vi "linx_stepper_control.vi"() -> ()   [LabVIEW 2017]
uses:
  <vilib>/MakerHub/LINX/Public/Peripherals/Digital/Digital Read 1 Chan.vi
  <vilib>/MakerHub/LINX/Public/Peripherals/Digital/Digital Read N Chans.vi
  <vilib>/MakerHub/LINX/Private/Local IO/LinxDigitalRead.vi
  <vilib>/MakerHub/LINX/Public/Utilities/Check Channel.vi
  <vilib>/MakerHub/LINX/Public/Utilities/Open Serial.vi
  <vilib>/MakerHub/LINX/Private/Utilties/Generate Error.vi
  <vilib>/MakerHub/LINX/LMH-LINX.lvlib
panel:
  out "position":sgl[unit] format="%#.6g"
  in  "home stepper":bool
  in  "error in (no error)":errorcluster
  in  "MG17Motor":refnum<k7>(container)
  out "counter":dbl
  out "up/down/same":i32
  out "Response encoder signed long":sgl
  out "Response i2c":u8[](array[numeric])
  in  "Line 1":string
  in  "Line 0":string
  out "step size":dbl
  out "DI Value":bool
  in  "stop":bool
  out "Response encoder":u8[](array[numeric])
  in  "Timeout (100 ms)":i32=100
  in  "Serial Port":refnum<visa-resource-name>="COM4"
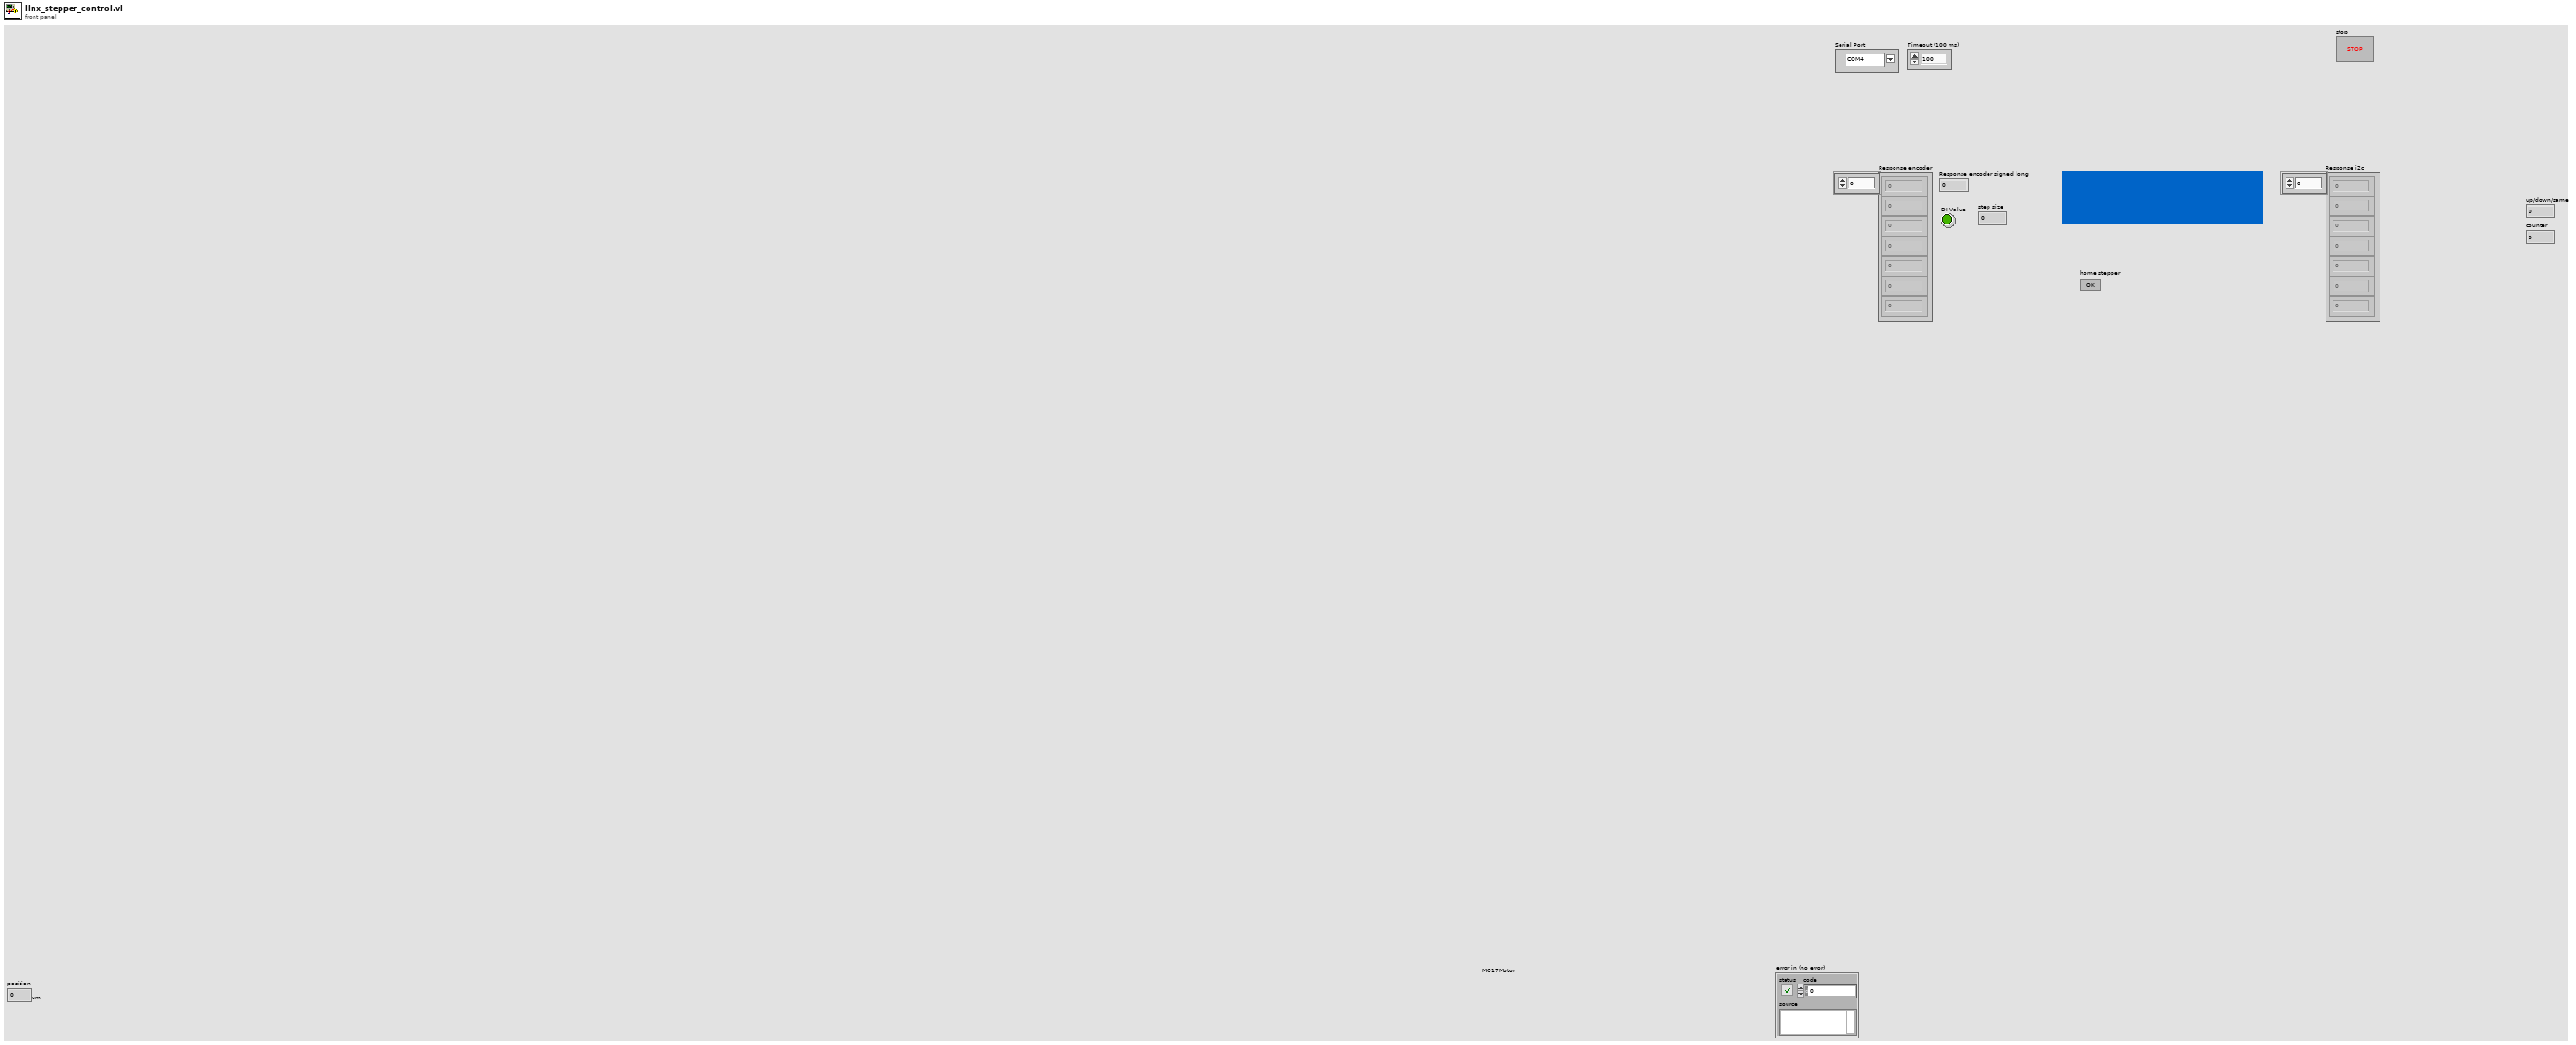
[diagram p1: front panel]
types:
  T1 = typedef "LMH-LINX.lvlib/LINX Ref.ctl" = cluster{"IO":T2, "Interface":T3, "LINX Device Config":T4}
  T2 = typedef "LMH-LINX.lvlib/Platform.ctl" = enum16{"Remote", "Local"}
  T3 = typedef "LMH-LINX.lvlib/Interface.ctl" = enum16{"Serial", "TCP"}
  T4 = typedef "LMH-LINX.lvlib/Device.lvlib/LINX Device Config.ctl" = cluster{"Interface":T3, "COM Port":refnum<visa-resource-name>, "TCP Configuration":T5, "Device Family":u8, "Device ID":u8, "Device Name":string, "TCP Ref":refnum<k5>, "Channels":T6}
  T5 = typedef "LMH-LINX.lvlib/Device.lvlib/TCP Config.ctl" = cluster{"IP Address":string, "Port":u16}
  T6 = typedef "LMH-LINX.lvlib/Channels.ctl" = cluster{"DI":u8[], "DO":u8[], "AI":u8[], "AO":u8[], "PWM":u8[], "QE":u8[], "UART":u8[], "I2C 2":u8[], "SPI":u8[], "CAN":u8[], "Servo":u8[], "AI Ref (V)":dbl, "AI Resolution (Bits)":u8, "AO Ref (V)":dbl, "AO Resolution (Bits)":u8}
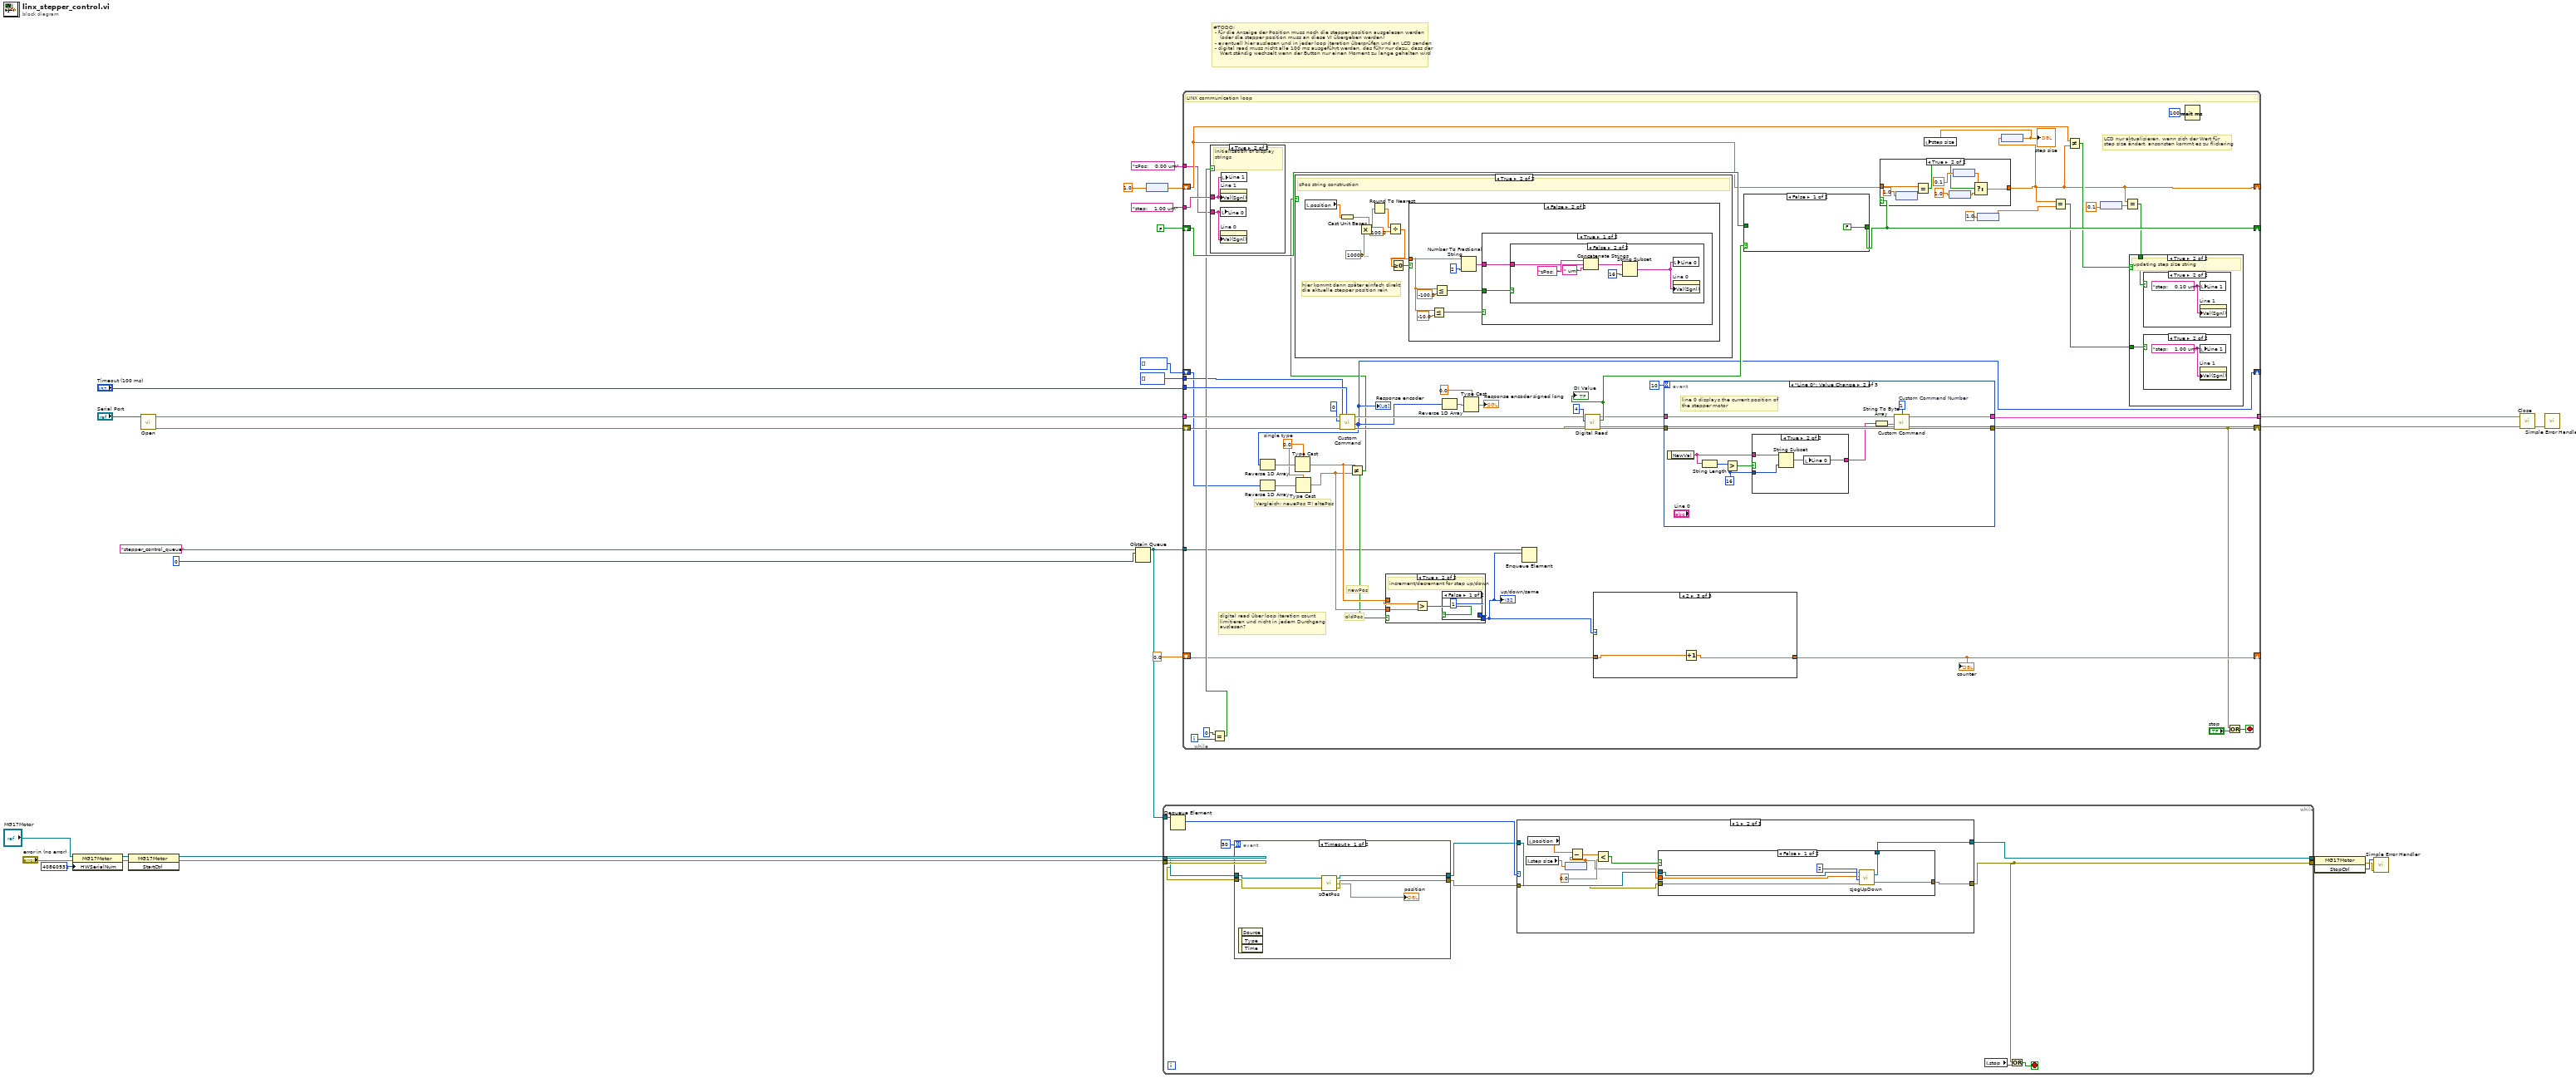
[diagram p0: block diagram]
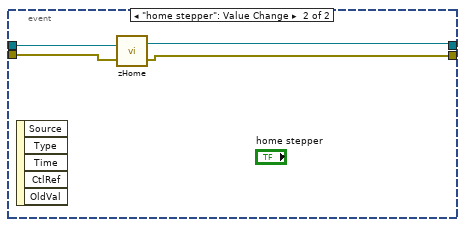
[diagram p2: hidden frame]
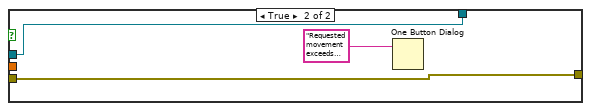
[diagram p4: hidden frame]
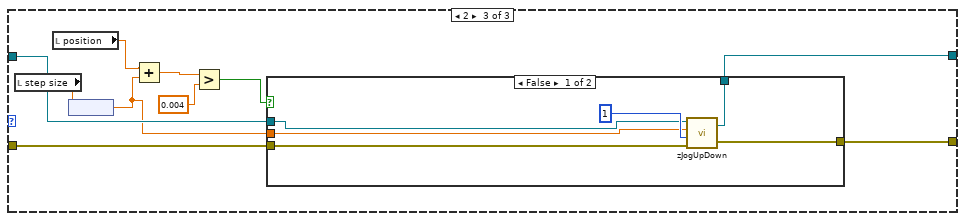
[diagram p5: hidden frame]
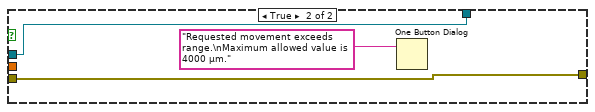
[diagram p6: hidden frame]
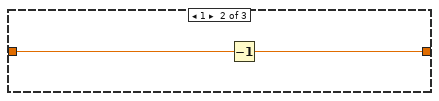
[diagram p8: hidden frame]
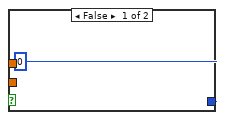
[diagram p9: hidden frame]
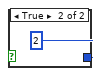
[diagram p10: hidden frame]
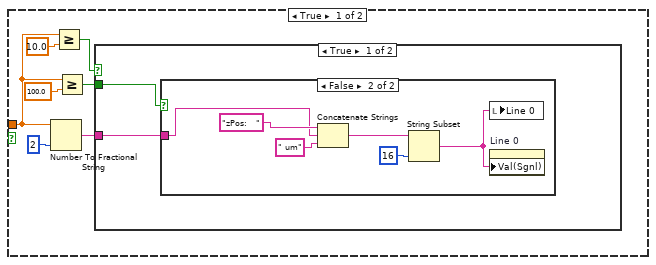
[diagram p12: hidden frame]
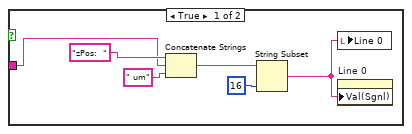
[diagram p13: hidden frame]
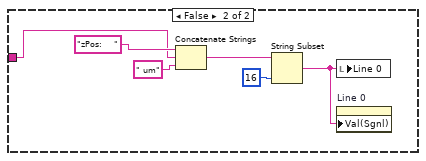
[diagram p14: hidden frame]
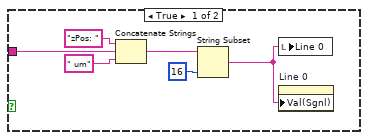
[diagram p15: hidden frame]
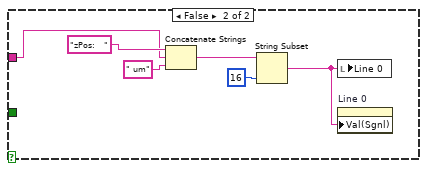
[diagram p16: hidden frame]
diagram:
  # "#TODO:\n - für die Anzeige der Position muss noch die stepper position ausgelesen werden\n    (oder die stepper position muss an diese VI übergeben werden)\n - eventuell hier auslesen und in jeder loop iteration überprüfen und an LCD senden\n - digital read muss nicht alle 100 ms ausgeführt werden, das führ nur dazu, dass der \n    Wert ständig wechselt wenn der Button nur einen Moment zu lange gehalten wird"
  n1 = property class="MG17Motor"(reference="MG17Motor", error in="error in (no error)", "HWSerialNum"=40860931) -> (reference out=w16:refnum<k7>, error out=w13:errorcluster)
  n2 = invoke class="MG17Motor" method="StartCtrl"(reference=w16, error in=w13) -> (reference out=w11:refnum<k7>, error out=w10:errorcluster)  [unwired: 1 in, 1 out]
  n3 = call-poly <vilib>:"Open.vi"("Serial Port"="Serial Port") -> ("Error Out"=w28:errorcluster, "LINX Resource"=w27:T1)  [unwired: 8 in, 1 out]
  n4 = Obtain Queue(name (unnamed)="stepper_control_queue", element data type=0) -> (queue out=w3:refnum<queue>)  [unwired: 3 in, 2 out]
  n5 = node(1.0) -> (w1:dbl[unit])
  n6 = while {
    tunnel: w11 -> [w37]
    tunnel: w10 -> [w36]
    tunnel: [w33] -> w9
    tunnel: [w32] -> w8
    tunnel: w3 -> [w39]
    stop <- w40 stop-if-true
    n7 = Dequeue Element(queue=w39) -> (element=w38:i32)  [unwired: 2 in, 3 out]
    n8 = event shown="[0] Timeout" {
      selector: _ -> [_ _]
      dyn-events: _ -> [_ _]
      timeout: 50 -> [_ _]
      tunnel: w37 -> [w45 w49]
      tunnel: w36 -> [w44 w46]
      tunnel: [w43 w48] -> w35
      tunnel: [w42 w47] -> w34
      event Timeout {
        n9 = event-data() -> ()  [unwired: 1 in, 3 out]
        n10 = call "zGetPos.vi"("error in (no error)"=w44, "reference in"=w45) -> ("error out"=w42:errorcluster, "position"=→"position":sgl[unit], "reference out"=w43:refnum<k7>)  [unwired: 1 in]
      }
      event "home stepper": Value Change {
        n11 = event-data() -> ()  [unwired: 1 in, 5 out]
        n12 = call "zHome.vi"("error in"=w46, "reference in"=w49) -> ("error out"=w47:errorcluster, "reference out"=w48:refnum<k7>)
      }
    }
    n13 = case shown="1" w38 {
      tunnel: w35 -> [w51 w55 w80]
      tunnel: w34 -> [w50 w54 w79]
      tunnel: [w51 w52 w78] -> w33
      tunnel: [w50 w53 w77] -> w32
      frame 0, Default {
      }
      frame 1 {
        n14 = local read "step size"() -> (w57:dbl)
        n15 = local read "position"() -> (w59:sgl[unit])
        n16 = node(w57) -> (w56:dbl[unit])
        n17 = Subtract(x=w59, y=w56) -> (x-y=w60:dbl[unit])
        n18 = Less?(x=w60, y=sgl[unit] 0.0) -> (x < y?=w58:bool)
        n19 = case shown="False" w58 {
          tunnel: [w67 w69] -> w53
          tunnel: w56 -> [w65 _]
          tunnel: w55 -> [w64 w68]
          tunnel: w54 -> [w63 w69]
          tunnel: [w62 w68] -> w52
          frame False {
            n20 = call "zJogUpDown.vi"("error in"=w63, "lJogDir"=2, "fStepSize"=w65, "reference in"=w64) -> ("error out"=w67:errorcluster, "reference out"=w62:refnum<k7>)
          }
          frame True {
            n21 = One Button Dialog(message="Requested movement exceeds range.\nMinimum allowed value is 0 µm.") -> ()  [unwired: 1 in, 1 out]
          }
        }
      }
      frame 2 {
        n22 = local read "step size"() -> (w72:dbl)
        n23 = local read "position"() -> (w73:sgl[unit])
        n24 = node(w72) -> (w71:dbl[unit])
        n25 = Add(x=w73, y=w71) -> (x+y=w75:dbl[unit])
        n26 = Greater?(x=w75, y=dbl[unit] 0.004) -> (0:w74:bool)
        n27 = case shown="False" w74 {
          tunnel: [w86 w88] -> w77
          tunnel: w71 -> [w81 _]
          tunnel: w80 -> [w84 w87]
          tunnel: w79 -> [w83 w88]
          tunnel: [w82 w87] -> w78
          frame False {
            n28 = call "zJogUpDown.vi"("error in"=w83, "lJogDir"=1, "fStepSize"=w81, "reference in"=w84) -> ("error out"=w86:errorcluster, "reference out"=w82:refnum<k7>)
          }
          frame True {
            n29 = One Button Dialog(message="Requested movement exceeds range.\nMaximum allowed value is 4000 µm.") -> ()  [unwired: 1 in, 1 out]
          }
        }
      }
    }
    n30 = local read "stop"() -> (w30:bool)
    n31 = Or(x=w32, y=w30) -> (x .or. y?=w40:bool)
  }
  n32 = while {
    tunnel: "Timeout (100 ms)" -> [w136]
    shift-right: [w96] -> w26
    shift-left: w28 -> [w138]
    shift-right: [w107] -> _
    shift-left: u8[] [] ("Response") -> [w104]
    tunnel: w27 -> [w137]
    tunnel: [w127] -> w25
    shift-right: [w91] -> _
    shift-left: w1 -> [w122]
    shift-right: [w130] -> _
    shift-left: FALSE -> [w131]
    tunnel: "step:    1,00 um" -> [w121]
    tunnel: "zPos:    0,00 um" -> [w113]
    tunnel: u8[] [] ("Data") -> [w112]
    shift-right: [w99] -> _
    shift-left: 0.0 -> [w100]
    tunnel: w3 -> [w98]
    i -> [w120]
    stop <- w134 stop-if-true
    w105 = sgl 0.0  # single type
    # "oldPos"
    # "newPos"
    # "Vergleich: neuePos =! altePos"
    # "LCD nur aktualisieren, wenn sich der Wert für\nstep size ändert, ansonsten kommt es zu flickering"
    # "digital read über loop iteration count \nlimitieren und nicht in jedem Durchgang \nauslesen?"
    # "LINX communication loop"
    n33 = Equal?(x=0, y=w120) -> (x = y?=w118:bool)
    n34 = case shown="True" w118 {
      tunnel: w121 -> [_ w214]
      tunnel: w113 -> [_ w213]
      frame False {
      }
      frame True {
        # "initialization of display strings"
        n35 = property on="Line 1" class="Str"("Val(Sgnl)"=w214) -> ()  [unwired: 2 in, 2 out]
        n36 = local write "Line 0"(w213) -> ()
        n37 = property on="Line 0" class="Str"("Val(Sgnl)"=w213) -> ()  [unwired: 2 in, 2 out]
        n38 = local write "Line 1"(w214) -> ()
      }
    }
    n39 = Reverse 1D Array(array=w104) -> (reversed array=w106:u8[])
    n40 = Type Cast(type=w105, x=w106) -> (*(type *) &x=w102:sgl)
    n41 = call <vilib>:"Custom Command.vi"("Timeout (100 ms)"=w136, "Error In"=w138, "Data"=w112, "Custom Command Number"=u16 0, "LINX Resource"=w137) -> ("Error Out"=w116:errorcluster, "Response"=w107:u8[], "LINX Resource"=w117:T1)  [unwired: 3 in, 1 out]
    "Response encoder" <- w107
    n42 = Reverse 1D Array(array=w107) -> (reversed array=w108:u8[])
    n43 = Type Cast(type=w105, x=w108) -> (*(type *) &x=w103:sgl)
    n44 = Not Equal?(x=w103, y=w102) -> (x != y?=w101:bool)
    n45 = case shown="True" w101 {
      frame False {
      }
      frame True {
        # "hier kommt dann später einfach direkt\ndie aktuelle stepper position rein"
        # "zPos string construction"
        n46 = local read "position"() -> (w157:sgl[unit])
        n47 = Cast Unit Bases(0:w157) -> (2:w155:sgl)  [unwired: 1 in]
        n48 = Multiply(x=w155, y=sgl 100000000.0) -> (x*y=w154:sgl)
        n49 = Round To Nearest(number=w154) -> (nearest integer value=w153:sgl)
        n50 = Divide(x=w153, y=sgl 100.0) -> (x/y=w151:sgl)
        n51 = Greater Or Equal To 0?(x=w151) -> (x >= 0?=w158:bool)
        n52 = case shown="False" w158 {
          tunnel: w151 -> [w159 w188]
          frame True {
            n53 = Number To Fractional String(number=w159, precision (6)=i16 2) -> (F-format string=w160:string)  [unwired: 2 in]
            n54 = Greater Or Equal?(x=w159, y=sgl 10.0 ("x")) -> (x >= y?=w165:bool)
            n55 = Greater Or Equal?(x=w159, y=sgl 100.0 ("x")) -> (x >= y?=w162:bool)
            n56 = case shown="True" w165 {
              tunnel: w160 -> [w167 w180]
              tunnel: w162 -> [w166 _]
              frame True {
                n57 = case shown="False" w166 {
                  tunnel: w167 -> [w168 w174]
                  frame True {
                    n58 = Concatenate Strings("zPos:  ", w168, " um") -> (w172:string)
                    n59 = String Subset(string=w172, length (rest)=16 ("length (rest)")) -> (substring=w171:string)  [unwired: 1 in]
                    n60 = local write "Line 0"(w171) -> ()
                    n61 = property on="Line 0" class="Str"("Val(Sgnl)"=w171) -> ()  [unwired: 2 in, 2 out]
                  }
                  frame False {
                    n62 = Concatenate Strings("zPos:   ", w174, " um") -> (w178:string)
                    n63 = String Subset(string=w178, length (rest)=16 ("length (rest)")) -> (substring=w177:string)  [unwired: 1 in]
                    n64 = local write "Line 0"(w177) -> ()
                    n65 = property on="Line 0" class="Str"("Val(Sgnl)"=w177) -> ()  [unwired: 2 in, 2 out]
                  }
                }
              }
              frame False {
                n66 = Concatenate Strings("zPos:    ", w180, " um") -> (w184:string)
                n67 = String Subset(string=w184, length (rest)=16 ("length (rest)")) -> (substring=w183:string)  [unwired: 1 in]
                n68 = local write "Line 0"(w183) -> ()
                n69 = property on="Line 0" class="Str"("Val(Sgnl)"=w183) -> ()  [unwired: 2 in, 2 out]
              }
            }
          }
          frame False {
            n70 = Less Or Equal?(x=w188, y=sgl -10.0 ("x")) -> (x <= y?=w192:bool)
            n71 = Less Or Equal?(x=w188, y=sgl -100.0 ("x")) -> (x <= y?=w190:bool)
            n72 = Number To Fractional String(number=w188, precision (6)=i16 2) -> (F-format string=w187:string)  [unwired: 2 in]
            n73 = case shown="True" w192 {
              tunnel: w190 -> [w194 _]
              tunnel: w187 -> [w193 w207]
              frame True {
                n74 = case shown="False" w194 {
                  tunnel: w193 -> [w195 w201]
                  frame True {
                    n75 = Concatenate Strings("zPos: ", w195, " um") -> (w199:string)
                    n76 = String Subset(string=w199, length (rest)=16 ("length (rest)")) -> (substring=w198:string)  [unwired: 1 in]
                    n77 = local write "Line 0"(w198) -> ()
                    n78 = property on="Line 0" class="Str"("Val(Sgnl)"=w198) -> ()  [unwired: 2 in, 2 out]
                  }
                  frame False {
                    n79 = Concatenate Strings("zPos:  ", w201, " um") -> (w205:string)
                    n80 = String Subset(string=w205, length (rest)=16 ("length (rest)")) -> (substring=w204:string)  [unwired: 1 in]
                    n81 = local write "Line 0"(w204) -> ()
                    n82 = property on="Line 0" class="Str"("Val(Sgnl)"=w204) -> ()  [unwired: 2 in, 2 out]
                  }
                }
              }
              frame False {
                n83 = Concatenate Strings("zPos:   ", w207, " um") -> (w211:string)
                n84 = String Subset(string=w211, length (rest)=16 ("length (rest)")) -> (substring=w210:string)  [unwired: 1 in]
                n85 = local write "Line 0"(w210) -> ()
                n86 = property on="Line 0" class="Str"("Val(Sgnl)"=w210) -> ()  [unwired: 2 in, 2 out]
              }
            }
          }
        }
      }
    }
    n87 = case shown="True" w101 {
      tunnel: w103 -> [_ w148]
      tunnel: w102 -> [_ w147]
      tunnel: [0 w145] -> w97
      frame False {
      }
      frame True {
        # "increment/decrement for step up/down"
        n88 = Greater?(x=w148, y=w147) -> (0:w146:bool)
        n89 = case shown="False" w146 {
          tunnel: [1 2] -> w145
          frame False {
          }
          frame True {
          }
        }
      }
    }
    "up/down/same" <- w97
    n90 = Reverse 1D Array(array=w107) -> (reversed array=w111:u8[])
    n91 = Type Cast(type=sgl 0.0, x=w111) -> (*(type *) &x=→"Response encoder signed long":sgl)
    n92 = Enqueue Element(queue=w98, element=w97) -> ()  [unwired: 2 in, 3 out]
    n93 = call-poly <vilib>:"Digital Read.vi"("Error In"=w116, "DI Channel"=u8 4, "LINX Resource"=w117) -> ("Error Out"=w128:errorcluster, "DI Value"=w132:bool, "LINX Resource"=w129:T1)  [unwired: 6 in]
    "DI Value" <- w132
    n94 = case shown="2" w97 {
      tunnel: w100 -> [w139 w141 w143]
      tunnel: [w139 w140 w142] -> w99
      frame 0, Default {
      }
      frame 1 {
        n95 = Decrement(x=w141) -> (x-1=w140:dbl)
      }
      frame 2 {
        n96 = Increment(x=w143) -> (x+1=w142:dbl)
      }
    }
    "counter" <- w99
    n97 = event shown="[1] \"Line 0\": Value Change" {
      selector: _ -> [_ _ _]
      dyn-events: _ -> [_ _ _]
      timeout: 10 -> [_ _ _]
      tunnel: w129 -> [w219 w227 w243]
      tunnel: [w219 w225 w241] -> w127
      tunnel: [w220 w224 w240] -> w96
      tunnel: w128 -> [w220 w226 w242]
      event Timeout {
        n98 = event-data() -> ()  [unwired: 1 in, 1 out]
      }
      event "Line 0": Value Change {
        w221 = u16 1  # Custom Command Number
        w228 = 16 ("y")
        # "line 0 displays the current position of \nthe stepper motor"
        n99 = event-data() -> ("NewVal"=w229:string)  [unwired: 1 in]
        n100 = String Length(string=w229) -> (length=w231:i32)
        n101 = Greater?(x=w231, y=w228) -> (0:w230:bool)
        n102 = case shown="True" w230 {
          tunnel: w229 -> [w232 w235]
          tunnel: w228 -> [_ w234]
          tunnel: [w232 w233] -> w222
          frame False {
          }
          frame True {
            n103 = String Subset(string=w235, length (rest)=w234) -> (substring=w233:string)  [unwired: 1 in]
            n104 = local write "Line 0"(w233) -> ()
          }
        }
        n105 = String To Byte Array(string=w222) -> (unsigned byte array=w223:u8[])
        n106 = call <vilib>:"Custom Command.vi"("Error In"=w226, "Data"=w223, "Custom Command Number"=w221, "LINX Resource"=w227) -> ("Error Out"=w224:errorcluster, "LINX Resource"=w225:T1)  [unwired: 4 in, 2 out]
      }
      event "Line 1": Value Change {
        w237 = u16 2  # Custom Command Number
        w244 = 16 ("y")
        # "line 1 displays the current step size"
        n107 = event-data() -> ("NewVal"=w245:string)  [unwired: 1 in]
        n108 = String Length(string=w245) -> (length=w247:i32)
        n109 = Greater?(x=w247, y=w244) -> (0:w246:bool)
        n110 = case shown="False" w246 {
          tunnel: w245 -> [w248 w251]
          tunnel: w244 -> [_ w250]
          tunnel: [w248 w249] -> w238
          frame False {
          }
          frame True {
            n111 = String Subset(string=w251, length (rest)=w250) -> (substring=w249:string)  [unwired: 1 in]
            n112 = local write "Line 1"(w249) -> ()
          }
        }
        n113 = String To Byte Array(string=w238) -> (unsigned byte array=w239:u8[])
        n114 = call <vilib>:"Custom Command.vi"("Error In"=w242, "Data"=w239, "Custom Command Number"=w237, "LINX Resource"=w243) -> ("Error Out"=w240:errorcluster, "Response"=→"Response i2c":u8[], "LINX Resource"=w241:T1)  [unwired: 4 in, 1 out]
      }
    }
    n115 = case shown="False" w132 {
      tunnel: w131 -> [_ w258]
      tunnel: [FALSE w255] -> w130
      frame False {
      }
      frame True {
        n116 = Equal?(x=w258, y=FALSE) -> (x = y?=w257:bool)
        n117 = Select(t=TRUE, s=w257, f=FALSE) -> (s? t:f=w255:bool)
      }
    }
    n118 = case shown="True" w130 {
      tunnel: [w259 w268] -> w91
      tunnel: w122 -> [w259 w267]
      frame False {
      }
      frame True {
        n119 = node(1.0 ("y")) -> (w266:dbl[unit])
        n120 = Equal?(x=w267, y=w266) -> (x = y?=w260:bool)
        n121 = node(1.0 ("f")) -> (w261:dbl[unit])
        n122 = node(0.1 ("t")) -> (w262:dbl[unit])
        n123 = Select(t=w262, s=w260, f=w261) -> (s? t:f=w268:dbl[unit])
      }
    }
    n124 = node(1.0 ("y")) -> (w92:dbl[unit])
    n125 = node(w91) -> (w90:dbl)
    "step size" <- w90
    n126 = local write "step size"(w90) -> ()
    n127 = Equal?(x=w91, y=w92) -> (x = y?=w125:bool)
    n128 = Not Equal?(x=w122, y=w91) -> (x != y?=w123:bool)
    n129 = node(0.1 ("y")) -> (w94:dbl[unit])
    n130 = Equal?(x=w91, y=w94) -> (x = y?=w124:bool)
    n131 = case shown="True" w123 {
      tunnel: w125 -> [_ w216]
      tunnel: w124 -> [_ w215]
      frame False {
      }
      frame True {
        # "updating step size string"
        n132 = case shown="True" w215 {
          frame False {
          }
          frame True {
            w217 = "step:    0,10 um"
            n133 = local write "Line 1"(w217) -> ()
            n134 = property on="Line 1" class="Str"("Val(Sgnl)"=w217) -> ()  [unwired: 2 in, 2 out]
          }
        }
        n135 = case shown="True" w216 {
          frame False {
          }
          frame True {
            w218 = "step:    1,00 um"
            n136 = local write "Line 1"(w218) -> ()
            n137 = property on="Line 1" class="Str"("Val(Sgnl)"=w218) -> ()  [unwired: 2 in, 2 out]
          }
        }
      }
    }
    n138 = Wait (ms)(milliseconds to wait=u32 100) -> ()  [unwired: 1 out]
    n139 = Or(x=w96, y="stop") -> (x .or. y?=w134:bool)
  }
  n140 = invoke class="MG17Motor" method="StopCtrl"(reference=w9, error in=w8) -> (error out=w4:errorcluster, "StopCtrl"=w5:i32)  [unwired: 1 in, 1 out]
  n141 = call <vilib>:"Simple Error Handler.vi"("error code (no error:0)"=w5, "error in (no error)"=w4) -> ()  [unwired: 3 in, 5 out]
  n142 = call <vilib>:"Close.vi"("Error In"=w26, "LINX Resource"=w25) -> ("Error Out"=w22:errorcluster)  [unwired: 9 in]
  n143 = call <vilib>:"Simple Error Handler.vi"("error in (no error)"=w22) -> ()  [unwired: 4 in, 5 out]
